vi "ConfigError.vi"(8 "error in (no error)":errorcluster, 10 "Key":string, 11 "Section":string) -> (0 "error out":errorcluster)   [LabVIEW 2009]
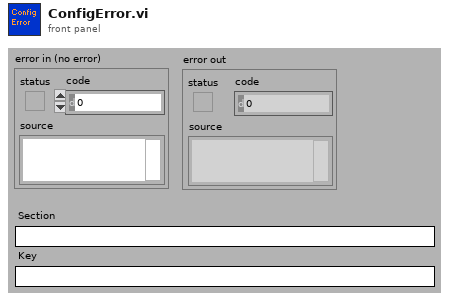
[diagram p1: front panel]
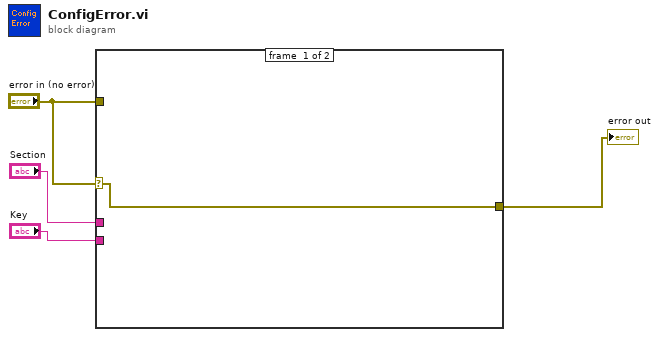
[diagram p0: block diagram]
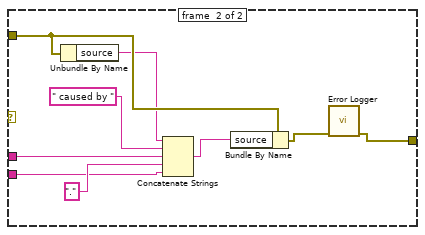
[diagram p2: hidden frame]
diagram:
  n1 = case shown="Error" "error in (no error)" {
    selector: "error in (no error)" -> [w5 _]
    tunnel: "error in (no error)" -> [_ w14]
    tunnel: "Section" -> [_ w11]
    tunnel: "Key" -> [_ w9]
    tunnel: [w5 w6] -> w2
    frame #0 {
    }
    frame #1 {
      n2 = Unbundle By Name(w14) -> ("source"=w13:string)
      n3 = Concatenate Strings(w13, " caused by " ("string"), w11, "." ("string"), w9) -> (w8:string)
      n4 = Bundle By Name(cluster=w14, "source"=w8) -> (w7:errorcluster)
      n5 = call "Error Logger.vi"("error in (no error)"=w7) -> ("error out"=w6:errorcluster)  [unwired: 1 in, 9 out]
    }
  }
  "error out" <- w2
